vi "Multiply.vi"() -> ()   [LabVIEW 2023]
panel:
  out "Out 3":dbl
  in  "y":dbl
  in  "x":dbl
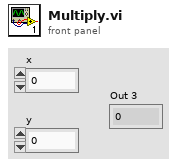
[diagram p1: front panel]
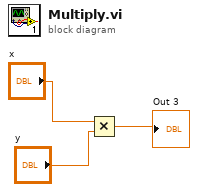
[diagram p0: block diagram]
diagram:
  n1 = Multiply(x="x", y="y") -> (x*y=→"Out 3":dbl)
